vi "main.vi"() -> ()   [LabVIEW 2019]
uses:
  <vilib>/regexp/Match Regular Expression.xnode
panel:
  in  "input string":string
  out "error out":errorcluster
  out "offset past match":i32
  out "after match":string
  out "whole match":string
  out "before match":string
  in  "multiline? (F)":bool
  in  "ignore case? (F)":bool
  in  "error in":errorcluster
  in  "offset (0)":i32
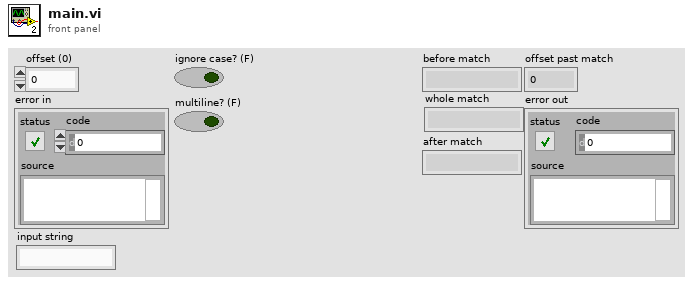
[diagram p1: front panel]
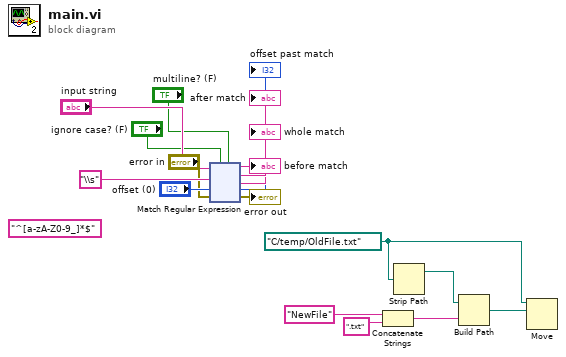
[diagram p0: block diagram]
diagram:
  w1 = path "C:/temp/OldFile.txt" ("path")
  (unwired) "^[a-zA-Z0-9_]*$" ("regular expression")
  n1 = xnode "Match Regular Expression"("input string"="input string", "regular expression"="\\s", "offset (0)"="offset (0)", "error in"="error in", "ignore case? (F)"="ignore case? (F)", "multiline? (F)"="multiline? (F)") -> ("before match"=→"before match":string, "whole match"=→"whole match":string, "after match"=→"after match":string, "offset past match"=→"offset past match":i32, "error out"=→"error out":errorcluster)
  n2 = Concatenate Strings("NewFile" ("name or relative path"), ".txt" ("string")) -> (w3:string)
  n3 = Strip Path(path=w1) -> (stripped path=w6:path)  [unwired: 1 out]
  n4 = Build Path(base path=w6, name or relative path=w3) -> (appended path=w2:path)
  n5 = Move(source path=w1, 10:w2) -> ()  [unwired: 3 in, 3 out]
